vi "Scene Item ID.vi"(8 "error in (no error)":errorcluster, 11 "RGetSceneItemID in":refnum<class "RGetSceneItemID.lvclass">) -> (0 "error out":errorcluster, 2 "Scene Item ID":i32, 3 "RGetSceneItemID out":refnum<class "RGetSceneItemID.lvclass">)   [LabVIEW 2022 SP3, in "obs-websocket-lv.lvlib" / "RGetSceneItemID.lvclass"]
uses:
  RGetSceneItemID.lvclass
  RGetSceneItemID.lvclass/RGetSceneItemID.ctl
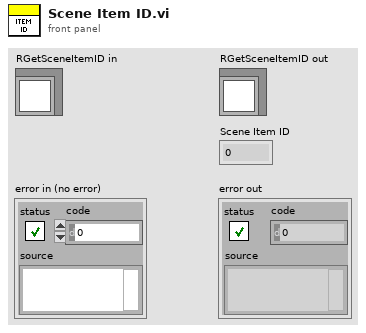
[diagram p1: front panel]
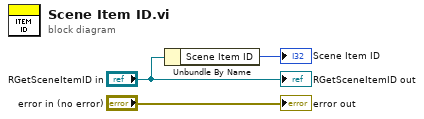
[diagram p0: block diagram]
diagram:
  n1 = Unbundle By Name("RGetSceneItemID in") -> ("Scene Item ID"=→"Scene Item ID":i32)
  "error out" <- "error in (no error)"
  "RGetSceneItemID out" <- "RGetSceneItemID in"
